vi "TagDB-Delete Single.vi"(8 "error in (no error)":errorcluster, 10 "tag":string, 11 "TagDB":T1) -> (0 "error out":errorcluster, 3 "TagDB(dup)":T1)   [LabVIEW 2017, in "TagDB.lvlib"]
uses:
  TagDB.lvlib
  Typedef/TagDB.ctl
  _Support/Error/_Build Error Cluster.vi
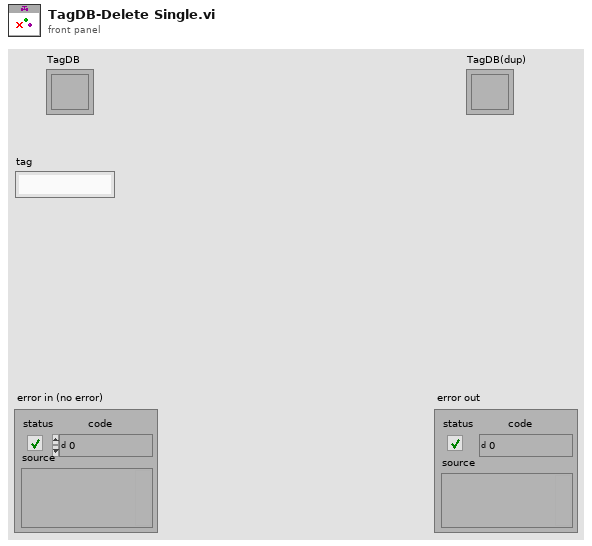
[diagram p1: front panel]
types:
  T1 = typedef "TagDB.lvlib/TagDB.ctl" = refnum<k1>
  T2 = typedef "TagDB.lvlib/tagdb-data.ctl" = cluster{"tag-map":variant, "timestamp-map":variant, "namecacher-map":variant, "DataTypeCacher-map":variant, "Tag Adding Lock?":bool, "Global Change Timestamp":timestamp, "Item Change Timestamp":timestamp, "name":string, "Global Change Flag":u64, "Item Change Flag":u64}
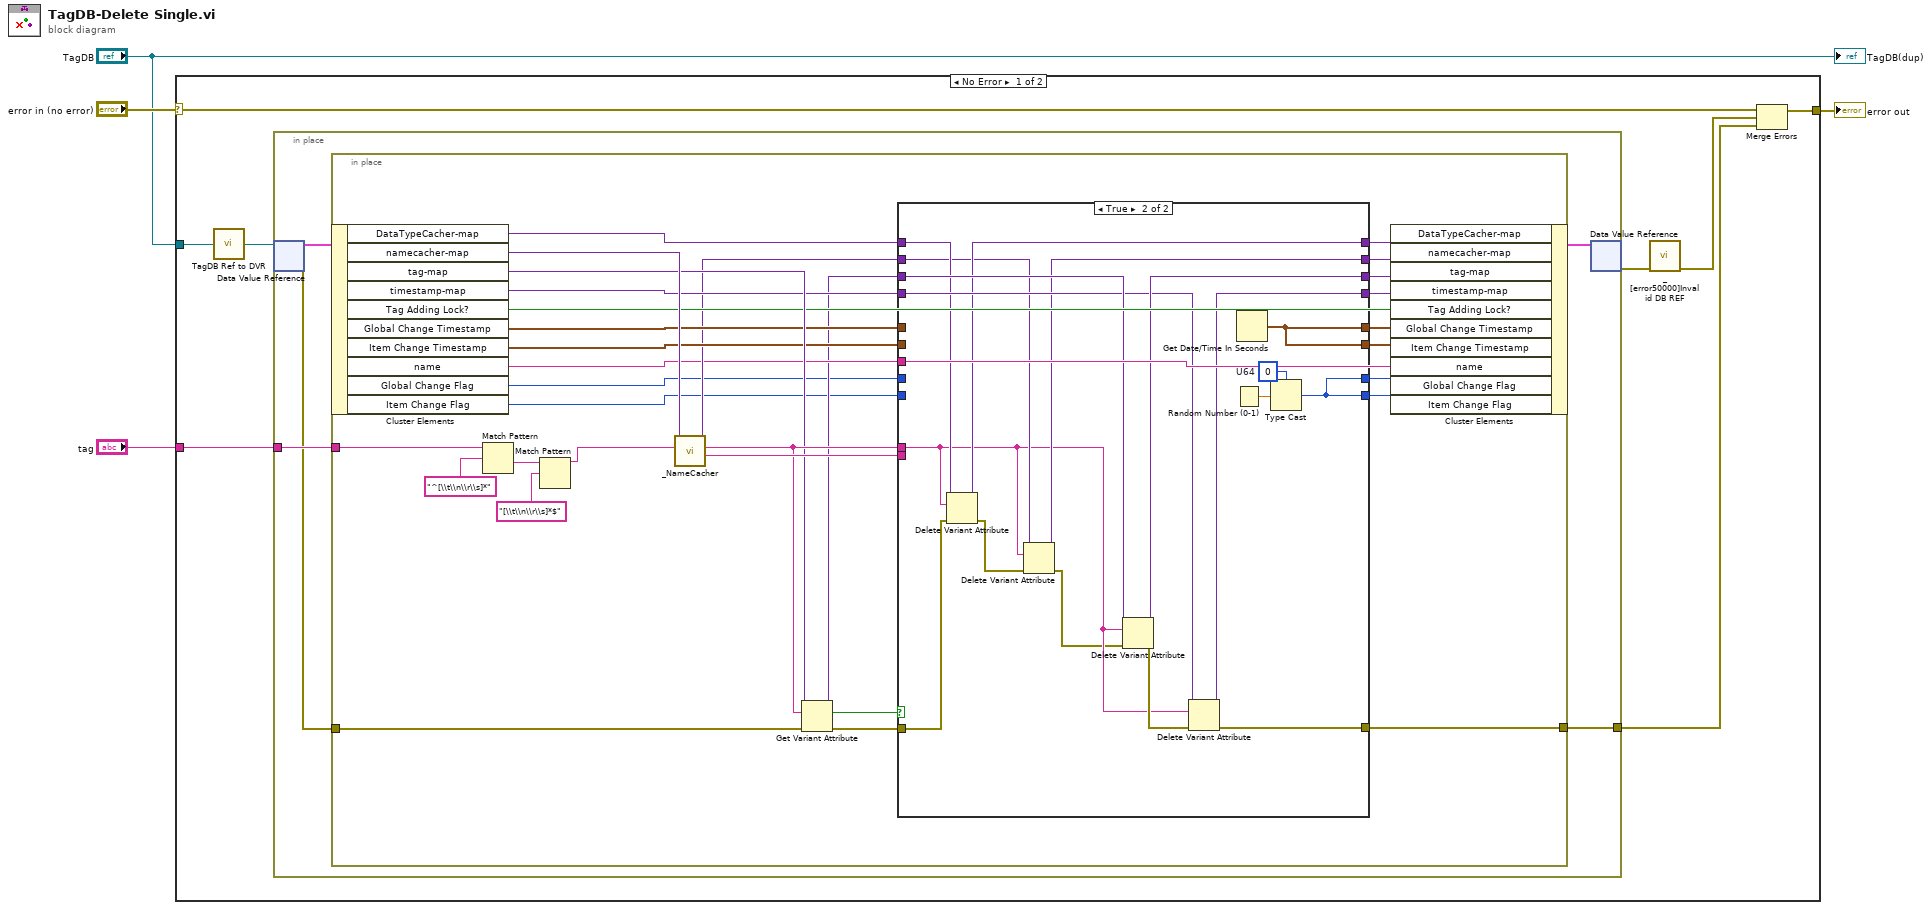
[diagram p0: block diagram]
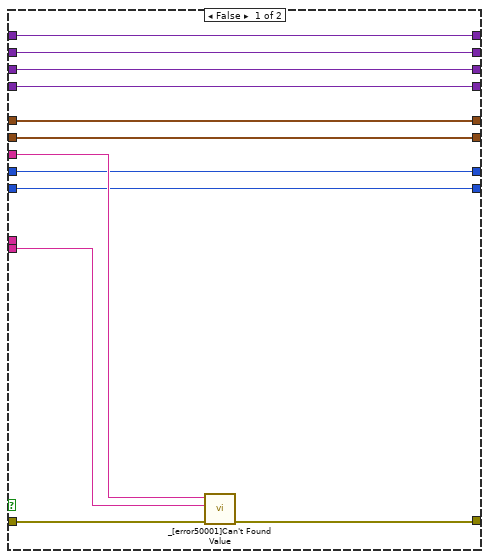
[diagram p2: hidden frame]
diagram:
  n1 = case shown="No Error" "error in (no error)" {
    selector: "error in (no error)" -> [w10 w79]
    tunnel: [w11 w79] -> w3
    tunnel: "TagDB" -> [w8 _]
    tunnel: "tag" -> [w6 _]
    frame No Error {
      n2 = call "TagDB Ref to DVR.vi"("TagDB"=w8) -> ("DVR"=w7:refnum<data-value>)  [unwired: 4 in]
      n3 = in-place "In Place Element Structure" {
        in-place-border: [w17] -> w12
        in-place-border: w6 -> [w16]
        n4 = in-place-dvr #1(w7) -> (w15:T2, w13:errorcluster)
        n5 = in-place {
          in-place-border: [w48] -> w17
          in-place-border: w16 -> [w19]
          in-place-border: w13 -> [w40]
          n6 = in-place-cluster #2(w15) -> ("DataTypeCacher-map"=w33:variant, "namecacher-map"=w45:variant, "tag-map"=w44:variant, "timestamp-map"=w43:variant, "Tag Adding Lock?"=w37:bool, "Global Change Timestamp"=w39:timestamp, "Item Change Timestamp"=w36:timestamp, "name"=w30:string, "Global Change Flag"=w25:u64, "Item Change Flag"=w24:u64)
          n7 = Match Pattern(string=w19, regular expression="^[\\t\\n\\r\\s]*") -> (after substring=w20:string)  [unwired: 1 in, 3 out]
          n8 = Match Pattern(string=w20, regular expression="[\\t\\n\\r\\s]*$") -> (before substring=w18:string)  [unwired: 1 in, 3 out]
          n9 = call "_NameCacher.vi"("key"=w18, "cacher"=w45) -> ("Raw name"=w47:string, "Key in lower case"=w46:string, "cacher out"=w31:variant)  [unwired: 7 in]
          n10 = Get Variant Attribute(Variant=w44, name=w46, error in=w40) -> (duplicate Variant=w28:variant, found=w27:bool, error out=w29:errorcluster)  [unwired: 1 in, 1 out]
          n11 = case shown="True" w27 {
            tunnel: [w53 w77] -> w48
            tunnel: w47 -> [w52 _]
            tunnel: w29 -> [w54 w64]
            tunnel: w28 -> [w60 w76]
            tunnel: [w60 w75] -> w42
            tunnel: w43 -> [w59 w73]
            tunnel: [w59 w74] -> w41
            tunnel: w46 -> [_ w67]
            tunnel: [w58 w72] -> w38
            tunnel: w39 -> [w58 _]
            tunnel: [w57 w72] -> w35
            tunnel: w36 -> [w57 _]
            tunnel: [w56 w70] -> w34
            tunnel: w33 -> [w56 w71]
            tunnel: [w55 w68] -> w32
            tunnel: w31 -> [w55 w69]
            tunnel: w30 -> [w51 _]
            tunnel: [w50 w61] -> w26
            tunnel: w25 -> [w50 _]
            tunnel: w24 -> [w49 _]
            tunnel: [w49 w61] -> w23
            frame False {
              n12 = call "_[error50001]Can't Found Value.vi"("error in (no error)"=w54, "db name"=w52, "value name"=w51) -> ("error out"=w53:errorcluster)  [unwired: 8 in]
            }
            frame True {
              w62 = u64 0  # U64
              n13 = Delete Variant Attribute(4:w64, 6:w67, 7:w71) -> (0:w66:errorcluster, 3:w70:variant)  [unwired: 1 out]
              n14 = Delete Variant Attribute(4:w66, 6:w67, 7:w69) -> (0:w65:errorcluster, 3:w68:variant)  [unwired: 1 out]
              n15 = Delete Variant Attribute(4:w65, 6:w67, 7:w76) -> (0:w78:errorcluster, 3:w75:variant)  [unwired: 1 out]
              n16 = Delete Variant Attribute(4:w78, 6:w67, 7:w73) -> (0:w77:errorcluster, 3:w74:variant)  [unwired: 1 out]
              n17 = Random Number (0-1)() -> (number: 0 to 1=w63:dbl)
              n18 = Get Date/Time In Seconds() -> (seconds since 1Jan1904=w72:timestamp)
              n19 = Type Cast(type=w62, x=w63) -> (*(type *) &x=w61:u64)
            }
          }
          n20 = in-place-cluster #2("DataTypeCacher-map"=w34, "namecacher-map"=w32, "tag-map"=w42, "timestamp-map"=w41, "Tag Adding Lock?"=w37, "Global Change Timestamp"=w38, "Item Change Timestamp"=w35, "name"=w30, "Global Change Flag"=w26, "Item Change Flag"=w23) -> (w14:T2)
        }
        n21 = in-place-dvr #1(w14) -> (w9:errorcluster)  [unwired: 1 out]
      }
      n22 = call "_[error50000]Invalid DB REF.vi"("error in (no error)"=w9) -> ("error out"=w5:errorcluster)  [unwired: 10 in]
      n23 = Merge Errors(w10, w5, w12) -> (w11:errorcluster)
    }
    frame Error {
    }
  }
  "error out" <- w3
  "TagDB(dup)" <- "TagDB"
